vi "DisconnectFromPannelAddressSpace.vi"(8 "error in (no error)":errorcluster, 11 "comms cluster":T1) -> (0 "error out":errorcluster)   [LabVIEW 2025]
doc: "Forces all panel outputs to zero/low and\nclears user from station (zeros station gate reg).\nIf block does not execute, gate will be held shut\nuntil either: local user reconnects then disconnects\nproperly, connection times out and gate auto-clears,\nor, stations is manually cleared from server \nmanagement.\n\nINPUTS:\n 1. comms cluster of:\n a) station reg start address\n b)16-bit modulo of local user IP\n c) MB comms line \n 2. comms error line\n\nOUTPUTS:\n 1. comms error line"
uses:
  <vilib>/Modbus/master/Modbus Master.lvclass
panel:
  # "Close comunication with MB server\n\nForces all panel outputs to zero/low and\nclears user from station (zeros station gate reg).\nIf block does not execute, gate will be held shut\nuntil either: local user reconnects then disconnects\nproperly, connection times out and gate auto-clears,\nor, stations is manually cleared from server \nmanagement.\n\nINPUTS:\n  1. comms cluster of:\n      a) station reg start address\n      b)16-bit modulo of local user IP\n      c) MB comms line \n   2. comms error line\n\nOUTPUTS:\n  1. comms error line"
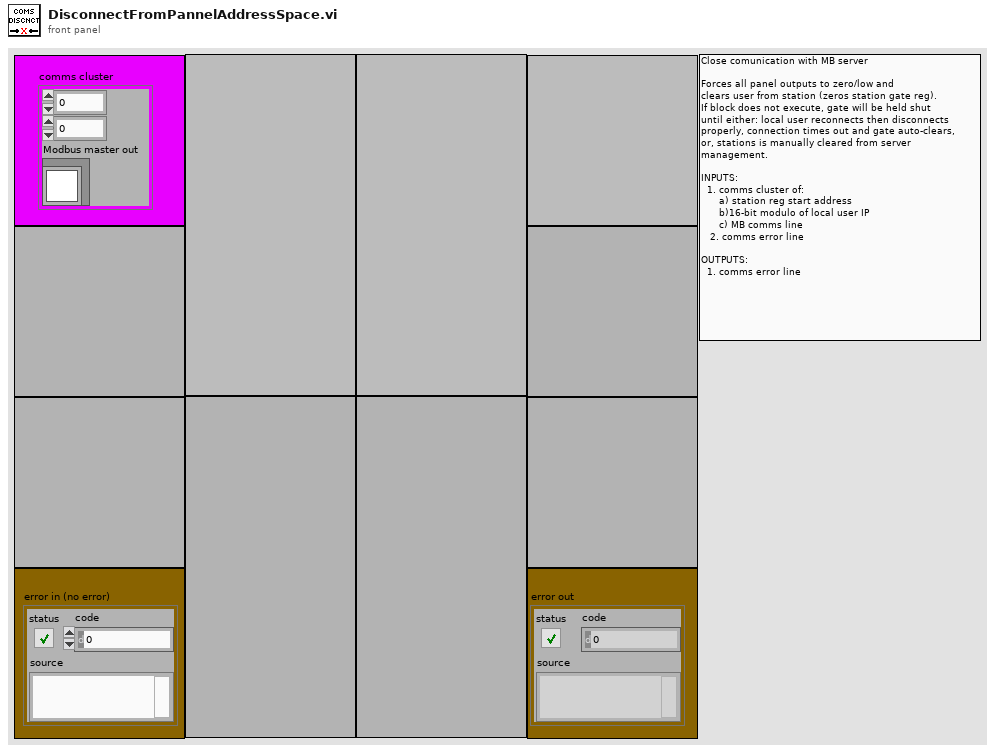
[diagram p1: front panel]
types:
  T1 = cluster{u16, u32, "Modbus master out":refnum<class "Modbus Master.lvclass">}
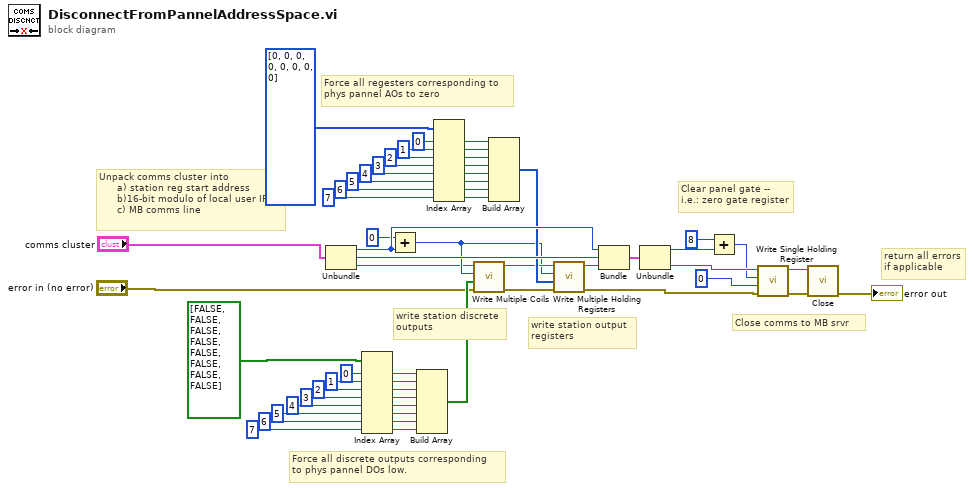
[diagram p0: block diagram]
diagram:
  # "write station discrete\noutputs"
  # "write station output\nregisters"
  # "return all errors\nif applicable"
  # "Close comms to MB srvr"
  # "Clear panel gate --\ni.e.: zero gate register"
  # "Force all regesters corresponding to\nphys pannel AOs to zero"
  # "Force all discrete outputs corresponding\nto phys pannel DOs low."
  # "Unpack comms cluster into\n      a) station reg start address\n      b)16-bit modulo of local user IP\n      c) MB comms line"
  n1 = Unbundle("comms cluster") -> (w46:u16, w45:u32, "Modbus master out"=w23:refnum<class "Modbus Master.lvclass">)
  n2 = Index Array(array=bool[] [FALSE, FALSE, FALSE, FALSE, FALSE, FALSE, FALSE, FALSE] ("Digital Write Values"), index #1=0 ("index"), index #2=1 ("index"), index #3=2 ("index"), index #4=3 ("index"), index #5=4 ("index"), index #6=5 ("index"), index #7=6 ("index"), index #8=7 ("index")) -> (element #1=w17:bool, element #2=w18:bool, element #3=w19:bool, element #4=w20:bool, element #5=w4:bool, element #6=w3:bool, element #7=w2:bool, element #8=w1:bool)
  n3 = Add(x=u16 0, y=w46) -> (x+y=w40:u16)
  n4 = Build Array(w17, w18, w19, w20, w4, w3, w2, w1) -> (w21:bool[])
  n5 = Index Array(array=i32[] [0, 0, 0, 0, 0, 0, 0, 0] ("Analog Write Values"), index #1=0 ("index"), index #2=1 ("index"), index #3=2 ("index"), index #4=3 ("index"), index #5=4 ("index"), index #6=5 ("index"), index #7=6 ("index"), index #8=7 ("index")) -> (element #1=w27:i32, element #2=w26:i32, element #3=w25:i32, element #4=w24:i32, element #5=w36:i32, element #6=w37:i32, element #7=w38:i32, element #8=w39:i32)
  n6 = call-dynamic "Write Multiple Coils.vi"("error in (no error)"="error in (no error)", "coil values"=w21, "starting address"=w40, "Modbus master in"=w23) -> ("error out"=w43:errorcluster, "Modbus master out"=w41:refnum<class "Modbus Master.lvclass">)  [unwired: 6 in]
  n7 = Build Array(w27, w26, w25, w24, w36, w37, w38, w39) -> (w42:i32[])
  n8 = call-dynamic "Write Multiple Holding Registers.vi"("error in (no error)"=w43, "holding register values"=w42, "starting address"=w40, "Modbus master in"=w41) -> ("error out"=w10:errorcluster, "Modbus master out"=w44:refnum<class "Modbus Master.lvclass">)  [unwired: 6 in]
  n9 = Bundle(w46, w45, "Modbus master out"=w44) -> (w9:T1)  [unwired: 1 in]
  n10 = Unbundle(w9) -> (w53:u16, "Modbus master out"=w55:refnum<class "Modbus Master.lvclass">)  [unwired: 1 out]
  n11 = Add(x=u16 8, y=w53) -> (x+y=w54:u16)
  n12 = call-dynamic "Write Single Holding Register.vi"("error in (no error)"=w10, "holding register value"=u16 0, "address"=w54, "Modbus master in"=w55) -> ("error out"=w51:errorcluster, "Modbus master out"=w50:refnum<class "Modbus Master.lvclass">)  [unwired: 6 in]
  n13 = call-dynamic "Close.vi"("error in (no error)"=w51, "Modbus master in"=w50) -> ("error out"=→"error out":errorcluster)  [unwired: 9 in]
